vi "Build.vi"(8 "error in (no error)":errorcluster, 10 "Transfer Group in":refnum<class "Transfer Group.lvclass">, 11 "Type Converter in":refnum<class "Simple Type Converter.lvclass">) -> (0 "error out":errorcluster, 2 "Transfer Group out":refnum<class "Transfer Group.lvclass">, 3 "Type Converter out":refnum<class "Simple Type Converter.lvclass">)   [LabVIEW 2017, in "DSF Core.lvlib" / "Simple Type Converter.lvclass"]
uses:
  Simple Type Converter.lvclass
  Classes/Transfer Group/Transfer Group.lvclass
  Simple Type Converter.lvclass/Simple Type Converter.ctl
  Convert String Block.vi
  VIs/Sizeof 1D.vi
  Classes/Buffer/Buffer.lvclass
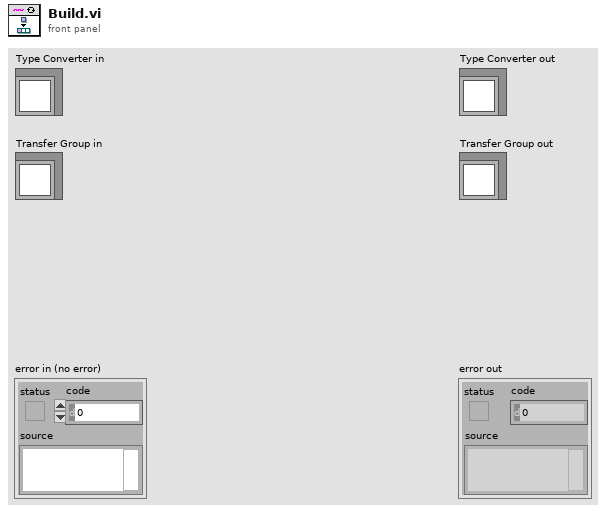
[diagram p1: front panel]
types:
  T1 = typedef "DSF Core.lvlib/Simple Type Converter.lvclass/Conversion.ctl" = cluster{"conversion blocks":T2[]}
  T2 = typedef "DSF Core.lvlib/Simple Type Converter.lvclass/Conversion Block.ctl" = cluster{"engine offset":u64, "engine data type":T3, "string offset":u64, "string data type":T3, "engine byte order":enum16{"big-endian, network order", "native, host order", "little-endian"}, "string byte order":enum16{"big-endian, network order", "native, host order", "little-endian"}, "count":u64}
  T3 = typedef "DSF Core.lvlib/DSF Data Type.ctl" = enum8{"Bool", "SGL", "DBL", "I8", "I16", "I32", "I64", "U8", "U16", "U32", "U64"}
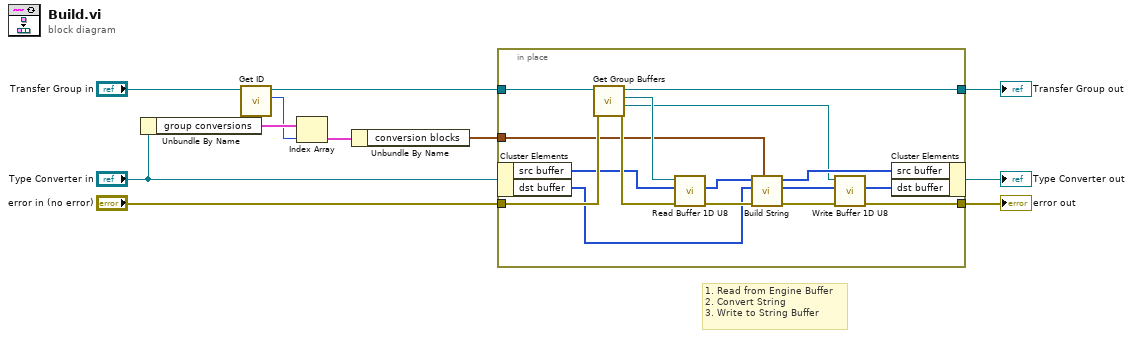
[diagram p0: block diagram]
diagram:
  # "1. Read from Engine Buffer\n2. Convert String\n3. Write to String Buffer"
  n1 = Unbundle By Name("Type Converter in") -> ("group conversions"=w10:T1[])
  n2 = call "Get ID.vi"("Transfer Group in"="Transfer Group in") -> ("id"=w7:i32, "Transfer Group out"=w3:refnum<class "Transfer Group.lvclass">)  [unwired: 9 in]
  n3 = Index Array(array=w10, index=w7) -> (element=w9:T1)
  n4 = Unbundle By Name(w9) -> ("conversion blocks"=w8:T2[])
  n5 = in-place {
    in-place-border: w8 -> [w14]
    in-place-border: [w22] -> w5
    in-place-border: "error in (no error)" -> [w21]
    in-place-border: w3 -> [w20]
    in-place-border: [w16] -> w2
    n6 = in-place-cluster #1("Type Converter in") -> ("src buffer"=w13:u8[], "dst buffer"=w18:u8[])
    n7 = call "Get Group Buffers.vi"("error in (no error)"=w21, "Transfer Group in"=w20) -> ("error out"=w19:errorcluster, "string Buffer"=w15:refnum<class "Buffer.lvclass">, "engine Buffer"=w17:refnum<class "Buffer.lvclass">, "Transfer Group out"=w16:refnum<class "Transfer Group.lvclass">)  [unwired: 6 in]
    n8 = call "Read Buffer 1D U8.vi"("error in (no error)"=w19, "dst array in"=w13, "Buffer in"=w17) -> ("error out"=w24:errorcluster, "dst array out"=w12:u8[])  [unwired: 5 in, 2 out]
    n9 = call "Build String.vi"("conversion blocks"=w14, "error in (no error)"=w24, "dst buffer in"=w18, "src buffer in"=w12) -> ("error out"=w23:errorcluster, "dst buffer out"=w27:u8[], "src buffer out"=w25:u8[])  [unwired: 5 in]
    n10 = call "Write Buffer 1D U8.vi"("error in (no error)"=w23, "src array in"=w27, "Buffer in"=w15) -> ("error out"=w22:errorcluster, "src array out"=w26:u8[])  [unwired: 5 in, 2 out]
    n11 = in-place-cluster #1("src buffer"=w25, "dst buffer"=w26) -> (→"Type Converter out":refnum<class "Simple Type Converter.lvclass">)
  }
  "error out" <- w5
  "Transfer Group out" <- w2
